vi "LVOBJ Set.vi"(8 "error in (no error)":errorcluster, 9 "Value":T1, 10 "JSON Path":string[](array[string]), 11 "Element in":T1) -> (0 "error out":errorcluster, 2 "Exists?":bool, 3 "Element out":T1)   [LabVIEW 2019, in "labview_json.lvlib"]
uses:
  labview_json.lvlib
  <vilib>/ErrorRing/Error Ring.xnode
  <vilib>/Utility/error.llb/Error Cluster From Error Code.vi
  Value Type.ctl
  Value.ctl
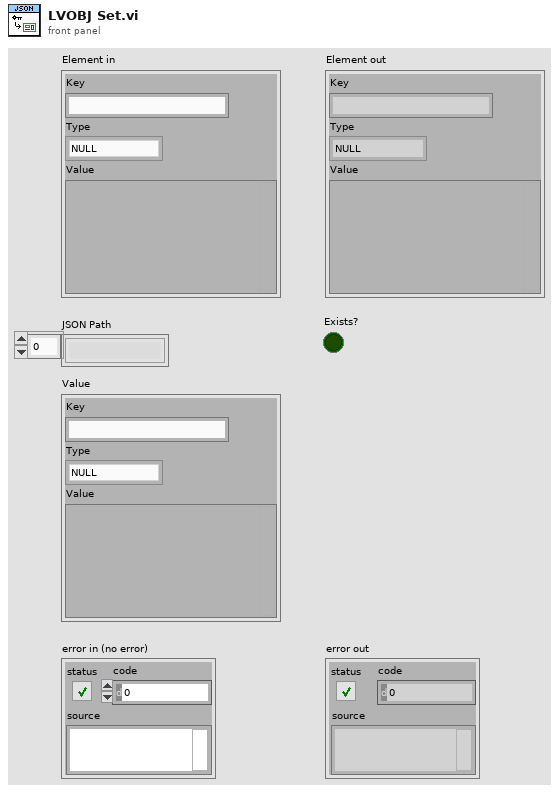
[diagram p1: front panel]
types:
  T1 = typedef "labview_json.lvlib/Value.ctl" = cluster{"Key":string, "Type":T2, "Value":variant}
  T2 = typedef "labview_json.lvlib/Value Type.ctl" = enum8{"NULL", "OBJECT", "ARRAY", "BOOL", "INT", "UINT", "FLOAT", "STRING"}
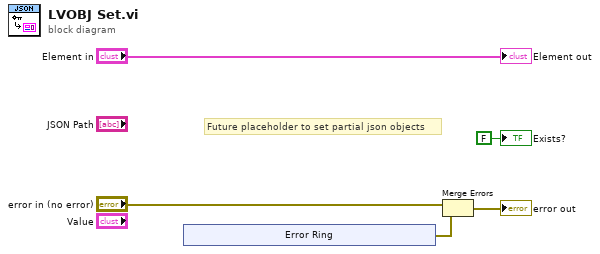
[diagram p0: block diagram]
diagram:
  # "Future placeholder to set partial json objects"
  n1 = xnode "Error Ring"() -> ("error out"=w2:errorcluster)
  n2 = Merge Errors("error in (no error)", w2) -> (→"error out":errorcluster)
  "Exists?" <- FALSE ("Exists?")
  "Element out" <- "Element in"
